vi "Transmitter_RSMA - 3 SC.vi"() -> ()   [LabVIEW 2022 SP3]
uses:
  <instrlib>/niUSRP/niUSRP Write Tx Data (CDB).vi
panel:
  in  "Beta/Alpha":dbl(slide)=0.17500000000000002 step=0.005 scale=0.0..1.0
  in  "Alpha":dbl(slide)=0.49999999999999994 step=0.005 scale=0.0..1.0
  in  "Tab Control":enum32{"USRP Parameters", "Transmission"}(tab)
  in  "USRP ControledParameters 2":T1={"Active Antenna"="TX1", "Gain (dB)"=0.0, "Carrier Frequency"=2400000000.0, "IQ Rate"=2000000.0, "Active Channel"="0"} {"IQ Rate" format="%#_6p"; "Carrier Frequency" format="%#_6p"; "Gain (dB)" format="%#_6f"}
  in  "Device selection":refnum<k15>="RIO0"
  in  "stop":bool
  out "Error out":errorcluster
  in  "Modulation parameter":T2
  out "Bits length":i32
  out "Bits length 2":i32
  out "Frame Duration":dbl format="%#_6p"
  out "Coerced Parameters":T3={"IQ Rate"=100000.0, "Carrier  Freq."=100000.0, "Gain"=0.0} {"Gain" format="%#_6f"; "Carrier  Freq." format="%#_6p"; "IQ Rate" format="%#_6p"}
  out "Transmitted Waveform":dbl[](graph)
  in  "Message 2":string="ptua. At vero eos et accusam et justo duo dolores et ea rebum. Stet clita kasd gubergren, no sea takimata sanctus est Lorem ipsum dolor sit amet. Lore"
  in  "Message 1":string="Lorem ipsum dolor sit amet, consetetur sadipscing elitr, sed diam nonumy eirmod tempor invidunt ut labore et dolore magna aliquyam erat, sed diam volu"
  in  "error in (no error)":errorcluster
  # "RSMA Transmitter"
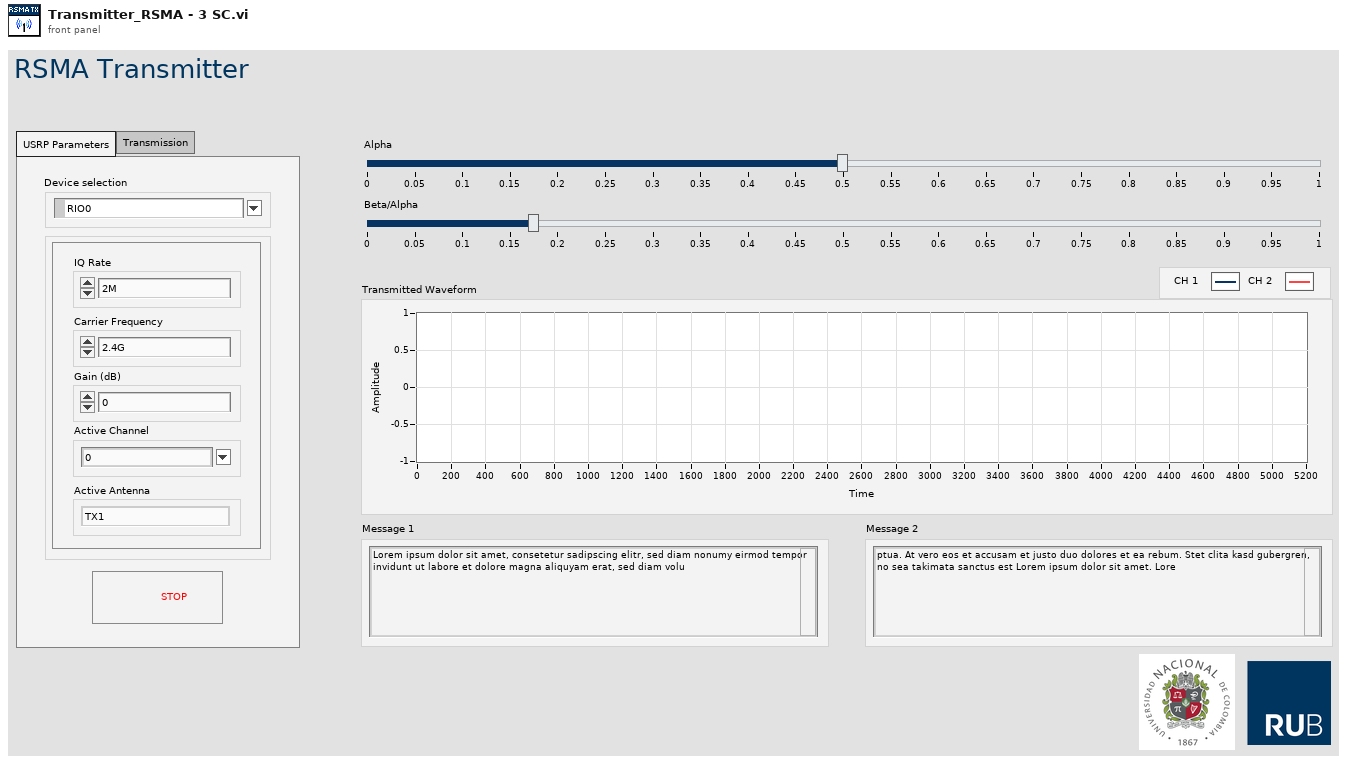
[diagram p1: front panel]
types:
  T1 = cluster{"Active Antenna":string, "Gain (dB)":dbl, "Carrier Frequency":dbl, "IQ Rate":dbl, "Active Channel":string}
  T2 = cluster{"Modulation type":enum16{"QPSK(4QAM)", "64QAM", "16QAM", "BPSK"}, "BCC rate (k/n)":enum16{"1/2", "2/3", "3/4"}}
  T3 = cluster{"IQ Rate":dbl, "Carrier  Freq.":dbl, "Gain":dbl}
  T4 = cluster{"coerced IQ rate":dbl, "coerced carrier frequency":dbl, "coerced gain":dbl}
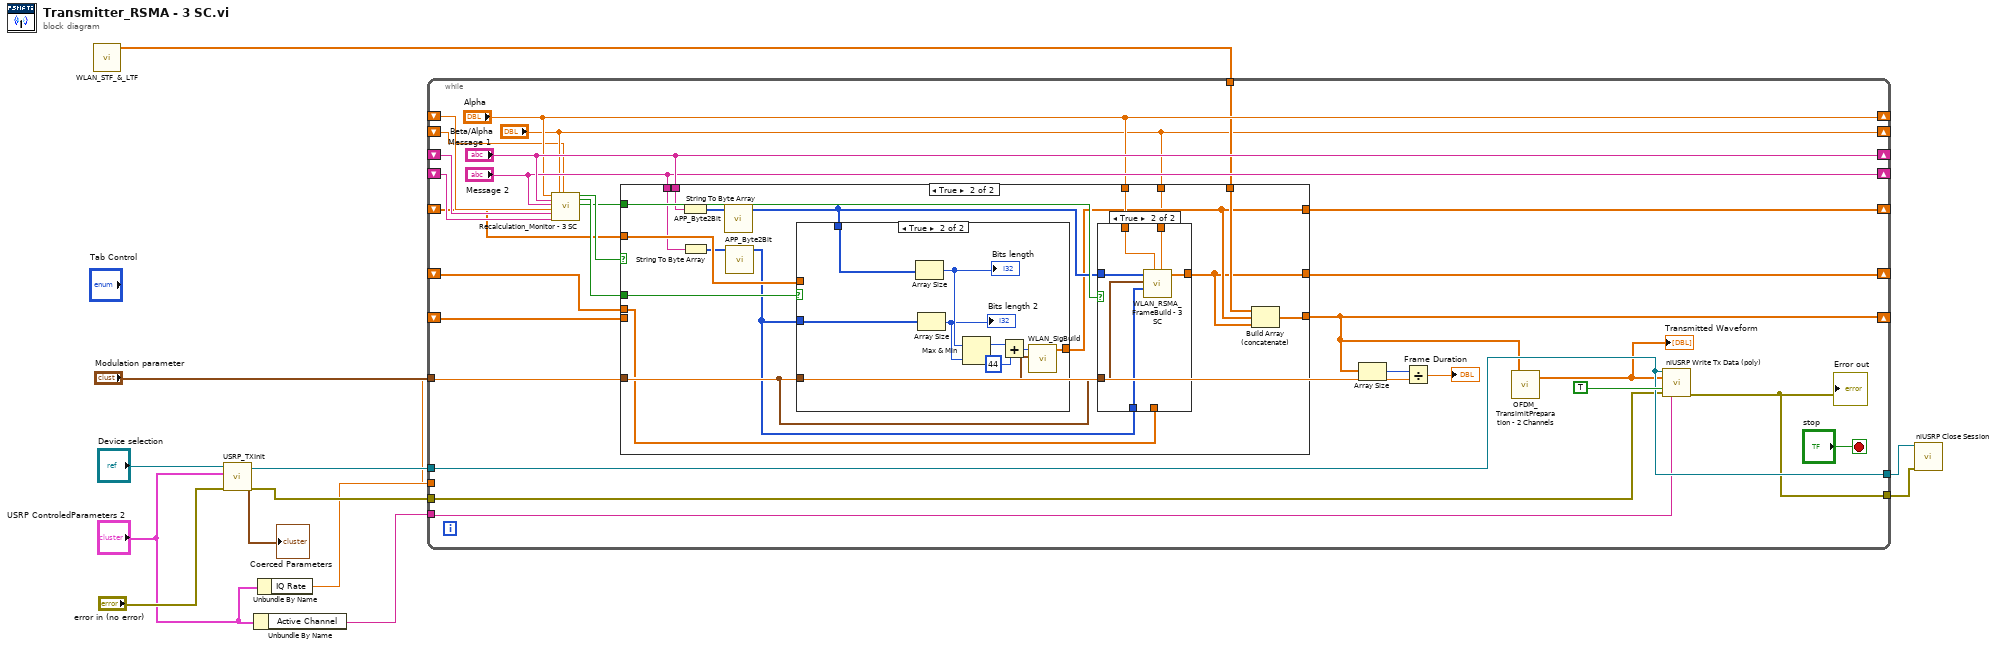
[diagram p0: block diagram]
diagram:
  n1 = call "WLAN_STF_&_LTF.vi"() -> ("STF & LTF"=w1:cdb[])  [unwired: 11 in]
  n2 = call "USRP_TXInit.vi"("device names"="Device selection", "USRP ControledParameters"="USRP ControledParameters 2", "error in (no error)"="error in (no error)") -> ("session handle out"=w11:refnum<k15>, "USRP CoercedParamters"=→"Coerced Parameters":T4, "error out"=w10:errorcluster)  [unwired: 5 in]
  n3 = Unbundle By Name("USRP ControledParameters 2") -> ("Active Channel"=w3:string)
  n4 = Unbundle By Name("USRP ControledParameters 2") -> ("IQ Rate"=w9:dbl)
  n5 = while {
    tunnel: w11 -> [w37]
    tunnel: w10 -> [w17]
    tunnel: w9 -> [w36]
    tunnel: [w37] -> w8
    tunnel: [w35] -> w7
    tunnel: w3 -> [w34]
    shift-right: ["Alpha"] -> _
    shift-left: _ -> [w33]
    shift-right: ["Message 1"] -> _
    shift-left: _ -> [w32]
    shift-right: ["Message 2"] -> _
    shift-left: _ -> [w31]
    tunnel: "Modulation parameter" -> [w25]
    shift-right: [w24] -> _
    shift-left: _ -> [w23]
    shift-right: [w21] -> _
    shift-left: _ -> [w20]
    tunnel: w1 -> [w19]
    shift-right: [w16] -> _
    shift-left: _ -> [w18]
    shift-right: ["Beta/Alpha"] -> _
    shift-left: _ -> [w13]
    stop <- "stop" stop-if-true
    n6 = call "Recalculation_Monitor - 3 SC.vi"("Alpha"="Alpha", "Message 1"="Message 1", "Message 2"="Message 2", "Alpha old"=w33, "Message 1 old"=w32, "Message 2 old"=w31, "Beta/Alpha"="Beta/Alpha", "Beta/Alpha old"=w13) -> ("Recalculate?"=w30:bool, "Recalculate SIG"=w29:bool, "Recalculate OFDM"=w28:bool)  [unwired: 9 in]
    n7 = case shown="True" w30 {
      tunnel: w29 -> [_ w61]
      tunnel: w28 -> [_ w60]
      tunnel: "Message 1" -> [_ w55]
      tunnel: "Message 2" -> [_ w56]
      tunnel: w25 -> [_ w52]
      tunnel: [w44 w48] -> w24
      tunnel: w23 -> [w44 w59]
      tunnel: "Alpha" -> [_ w51]
      tunnel: [w43 w47] -> w21
      tunnel: w20 -> [w43 w50]
      tunnel: w19 -> [_ w49]
      tunnel: [w42 w46] -> w16
      tunnel: w18 -> [w42 _]
      tunnel: "Beta/Alpha" -> [_ w45]
      frame False {
      }
      frame True {
        n8 = String To Byte Array(string=w55) -> (unsigned byte array=w57:u8[])
        n9 = String To Byte Array(string=w56) -> (unsigned byte array=w58:u8[])
        n10 = call "APP_Byte2Bit.vi"("input byte stream"=w57) -> ("output bit stream"=w53:i8[])  [unwired: 10 in]
        n11 = call "APP_Byte2Bit.vi"("input byte stream"=w58) -> ("output bit stream"=w54:i8[])  [unwired: 10 in]
        n12 = case shown="True" w61 {
          tunnel: w52 -> [_ w70]
          tunnel: [w69 w76] -> w48
          tunnel: w59 -> [w69 _]
          tunnel: w54 -> [_ w72]
          tunnel: w53 -> [_ w71]
          frame False {
          }
          frame True {
            n13 = Array Size(array=w71) -> (size(s)=w78:i32)
            "Bits length" <- w78
            n14 = Array Size(array=w72) -> (size(s)=w77:i32)
            "Bits length 2" <- w77
            n15 = Max & Min(x=w78, y=w77) -> (max(x,y)=w74:i32)  [unwired: 1 out]
            n16 = Add(x=w74, y=44) -> (x+y=w75:i32)
            n17 = call "WLAN_SigBuild.vi"("Data bit length"=w75, "Modulation parameter"=w70) -> ("symbols"=w76:cdb[])  [unwired: 7 in, 1 out]
          }
        }
        n18 = case shown="True" w60 {
          tunnel: w54 -> [_ w68]
          tunnel: w53 -> [_ w67]
          tunnel: w52 -> [_ w66]
          tunnel: w51 -> [_ w65]
          tunnel: [w62 w64] -> w47
          tunnel: w50 -> [w62 _]
          tunnel: w45 -> [_ w63]
          frame False {
          }
          frame True {
            n19 = call "WLAN_RSMA_FrameBuild - 3 SC.vi"("Beta/Alpha"=w63, "Alpha"=w65, "data in 2"=w68, "Modulation parameter"=w66, "data in"=w67) -> ("output array"=w64:cdb[])  [unwired: 5 in, 1 out]
          }
        }
        n20 = Build Array (concatenate)(w49, w48, w47) -> (w46:cdb[])
      }
    }
    n21 = Array Size(array=w16) -> (size(s)=w39:i32)
    n22 = Divide(x=w39, y=w36) -> (x/y=→"Frame Duration":dbl)
    n23 = call "OFDM_TransimitPreparation - 2 Channels.vi"("array"=w16) -> ("output array"=w15:cdb[])  [unwired: 8 in, 2 out]
    "Transmitted Waveform" <- w15
    n24 = call-poly <instrlib>:"niUSRP Write Tx Data (poly).vi"("session handle"=w37, "channel list"=w34, "data"=w15, "end of data?"=TRUE, "error in (no error)"=w17) -> ("error out"=w35:errorcluster)  [unwired: 9 in, 1 out]
    "Error out" <- w35
  }
  n25 = call <instrlib>:"niUSRP Close Session.vi"("session handle"=w8, "error in (no error)"=w7) -> ()  [unwired: 13 in, 1 out]
